vi "SPC_read_data_page.vi"(6 "DataBuffer":u16[](array[numeric]), 7 "First Page":i32 min=0 max=65535 step=1, 8 "Error In":errorcluster, 9 "Last Page":i32 min=0 max=65535 step=1, 10 "Module No":i16 min=0 max=7 step=1, 11 "DLL Path":path) -> (0 "Error Out":errorcluster, 2 "Module No":i16 min=0 max=7 step=1, 3 "DLL Path":path, 4 "Output Data":u16[](array[numeric]))   [LabVIEW 2019]
doc: "The procedure reads data from the pages of the SPC memory on module 'mod_no' defined by the parameters 'first_page' and 'last_page to the buffer 'data'. The procedure is used to read measurement results from the SPC memory.\nThe procedure is recommended when big amounts of SPC memory must be read as fast as possible, because it works much faster than calling in the loop the function SPC_read_data_block. Even the whole memory bank can be read in one call, when 'first_page' = 0 and 'last_page' = maxpage - 1.\nThe range of the parameters 'first_page' and 'last_page' depends on the actual configuration of the SPC memory (see SPC_configure_memory).\nTo provide correct access to the SPC memory it is required that the function SPC_configure_memory be used ( in normal operation modes) before the first call of SPC_read_data_page. This function also delivers the required information about the block/page structure of the SPC memory:\nlong max_block_no total number of blocks (=curves) in the memory ( memory bank for the SPC- 6x0/13x/15x/160)\nlong blocks_per_frame Number of blocks (=curves) per frame\nlong frames_per_page Number of frames per page\nlong maxpage max number of pages to use in a measurement\nlong block_length Number of 16-bits words per one block (curve)\nPlease make sure that the buffer 'data' be allocated with enough memory for \nblock_length * blocks_per_frame * frames_per_page * (last_page - first_page +1) 16-bit values.\n\n<b>Note:</b> This VI is set to execute as preallocated clone to improve performance when run in parallel loops for multi module setups.\n\ninfo@becker-hickl.com"
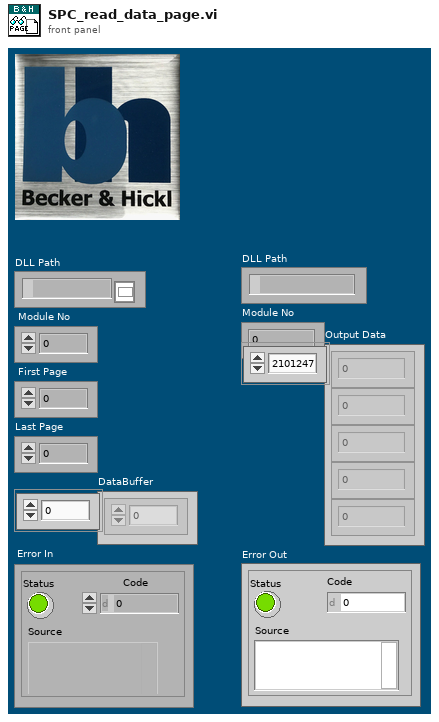
[diagram p1: front panel]
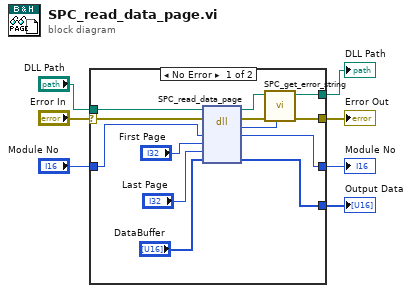
[diagram p0: block diagram]
diagram:
  n1 = case shown="No Error" "Error In" {
    selector: "Error In" -> [w18 w23]
    tunnel: [w15 w23] -> w7
    tunnel: "DLL Path" -> [w17 w22]
    tunnel: [w13 w22] -> w4
    tunnel: "Module No" -> [w11 w21]
    tunnel: [w10 w21] -> w2
    tunnel: [w8 _] -> w1
    frame No Error {
      n2 = dll-call lib="D:/spcm/lib/lab_view/lv10.0/spcm32.dll" fn="SPC_read_data_page"(path in=w17, error in=w18, "mod_no"=w11, "first_page"="First Page", "last_page"="Last Page", "data"="DataBuffer") -> (path out=w14:path, error out=w16:errorcluster, "return type"=w12:i16, "mod_no"=w10:i16, "data"=w8:u16[])  [unwired: 3 in]
      n3 = call "SPC_get_error_string.vi"("ErrorID"=w12, "Error In"=w16, "DLL Path"=w14) -> ("Error Out"=w15:errorcluster, "DLL Path"=w13:path)  [unwired: 6 in, 1 out]
    }
    frame Error {
    }
  }
  "DLL Path" <- w4
  "Error Out" <- w7
  "Module No" <- w2
  "Output Data" <- w1
